vi "Add Control to Cluster.vi"(7 "New Control Label":string, 8 "error in (no error)":errorcluster, 9 "Cluster ref in (owner)":refnum<vi>, 10 "Control ref in":refnum<vi>, 11 "Owning VI ref in":refnum<vi>) -> (0 "error out":errorcluster, 1 "Cluster ref out (owner)":refnum<vi>, 2 "Control ref out":refnum<vi>, 3 "Owning VI ref out":refnum<vi>)   [LabVIEW 2019, in "gRPC Scripting Tools.lvlib"]
uses:
  gRPC Scripting Tools.lvlib
  <vilib>/Utility/miscctls.llb/LVPositionTypeDef.ctl
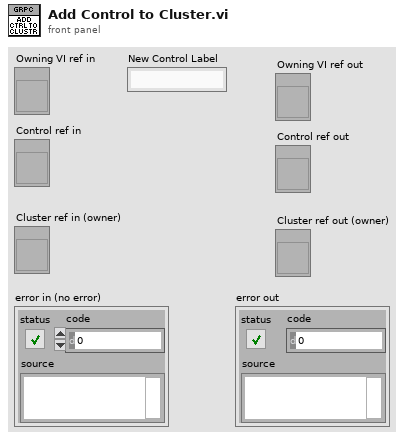
[diagram p1: front panel]
types:
  T1 = typedef "LVPositionTypeDef.ctl" = cluster{"Left":i32, "Top":i32}
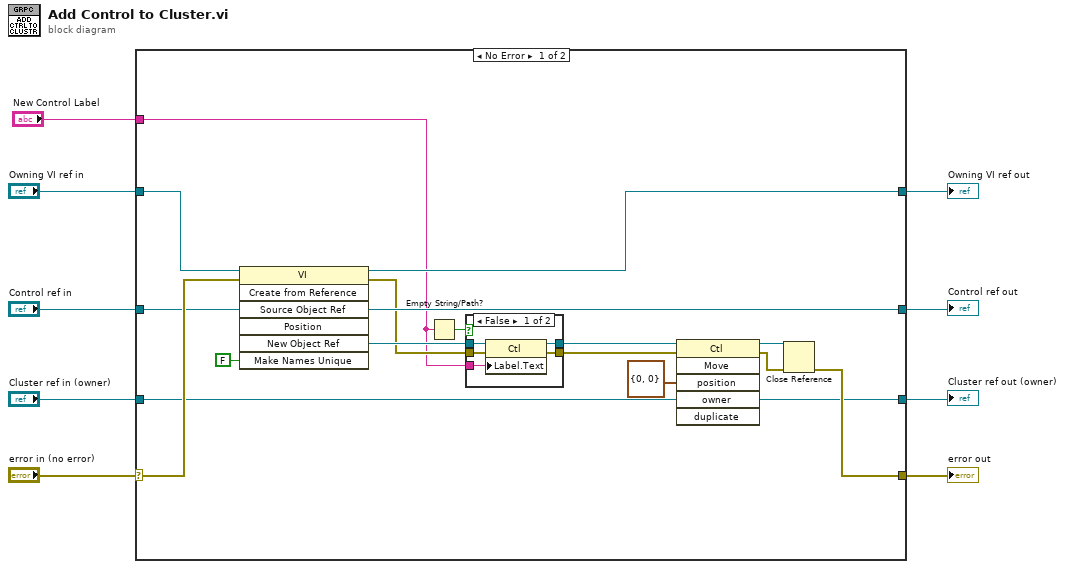
[diagram p0: block diagram]
diagram:
  n1 = case shown="No Error" "error in (no error)" {
    selector: "error in (no error)" -> [w18 w33]
    tunnel: [w25 w36] -> w9
    tunnel: "Owning VI ref in" -> [w24 w36]
    tunnel: "Control ref in" -> [w17 w35]
    tunnel: "Cluster ref in (owner)" -> [w16 w34]
    tunnel: [w19 w33] -> w5
    tunnel: [w17 w35] -> w3
    tunnel: [w16 w34] -> w2
    tunnel: "New Control Label" -> [w11 _]
    frame No Error {
      n2 = invoke class="VI" method="Create from Reference"(reference=w24, error in=w18, "Source Object Ref"=w17, "Make Names Unique"=FALSE ("Make Names Unique (F)")) -> (reference out=w25:refnum<vi>, error out=w13:errorcluster, "New Object Ref"=w15:refnum<vi>)  [unwired: 3 in, 4 out]
      n3 = Empty String/Path?(string/path=w11) -> (empty?=w10:bool)
      n4 = case shown="False" w10 {
        tunnel: w15 -> [w30 w32]
        tunnel: [w29 w32] -> w14
        tunnel: w11 -> [w28 _]
        tunnel: w13 -> [w27 w31]
        tunnel: [w26 w31] -> w12
        frame False {
          n5 = property class="Ctl"(reference=w30, error in=w27, "Label.Text"=w28) -> (reference out=w29:refnum<vi>, error out=w26:errorcluster)
        }
        frame True {
        }
      }
      n6 = invoke class="Ctl" method="Move"(reference=w14, error in=w12, "position"=T1 {"Left"=0, "Top"=0}, "owner"=w16) -> (reference out=w21:refnum<vi>, error out=w20:errorcluster)  [unwired: 2 in, 4 out]
      n7 = Close Reference(reference=w21, error in (no error)=w20) -> (error out=w19:errorcluster)
    }
    frame Error {
    }
  }
  "error out" <- w5
  "Owning VI ref out" <- w9
  "Control ref out" <- w3
  "Cluster ref out (owner)" <- w2
